vi "Eagle_FPGA Scanner Control.vi"() -> ()   [LabVIEW 2015]
uses:
  <vilib>/Platform/TimedLoop/XDataNode/timing_clust.ctl
  <vilib>/Platform/TimedLoop/XDataNode/nitl_modes.ctl
  <vilib>/Platform/TimedLoop/XDataNode/wakeup.ctl
  <vilib>/rvi/Emulation/niFpgaGetClockAttributes.vi
  <vilib>/rvi/Emulation/niFpgaSctlEmulationGetInTimedLoop.vi
  <vilib>/rvi/Emulation/niFpgaEmulationReportErrorSimple.vi
  <vilib>/rvi/eio/common/nirviEmuTemplateMethod_errors.vi
  <vilib>/rvi/Emulation/niFpgaProcessEmulError.vi
  <vilib>/rvi/Emulation/niFpgaCriticalErrorInLSC.vi
  <vilib>/rvi/FXPMathLib/FxpMul/XNode/nifxpmath_Multiplier.xnode
  <vilib>/eio/EIONode/EIONode.xnode
  <vilib>/rvi/FXPMathLib/FxpAdd/XNode/nifxpmath_Add.xnode
  <vilib>/Platform/TimedLoop/XDataNode/XDataNode.xnode
  <vilib>/rvi/FXPMathLib/sim/FxpSim.dll
  <vilib>/Platform/TimedLoop/XDataNode/XDNodeRunTimeDep.lvlib
  <vilib>/rvi/DataTransferAndStorage/Container/XNode/niFpgaContainer.xnode
  <vilib>/rvi/interface/RandomDataEmulation/nirviRandomDataFpgaMultiElementTemplate.vi
panel:
  in  "One Shot":bool
  in  "Illumination_Ena":bool
  out "Tmp Sens 2":fxp<+,18,3>
  out "Tmp Sens 1":fxp<+,18,3>
  out "X READ 2":fxp<+/-,20,5>
  out "Y READ 2":fxp<+/-,20,5>
  in  "Aim Ctrl":fxp<+,16,3>
  in  "V Range Ctrl":fxp<+,16,3>
  in  "H Range Ctrl":fxp<+,16,3>
  in  "Red Dots Ctrl":fxp<+,16,3>
  in  "LED Ring Ctrl":fxp<+,16,3>
  in  "Y Servo Ena":fxp<+,16,3>
  in  "X Servo Ena":fxp<+,16,3>
  in  "Manual VY":fxp<+/-,20,5>
  in  "Manual VX":fxp<+/-,20,5>
  in  "VX OFFS":fxp<+/-,20,5>
  in  "VY OFFS":fxp<+/-,20,5>
  out "X CMD IND":fxp<+/-,20,5>
  out "Y CMD IND":fxp<+/-,20,5>
  in  "Manual":bool
  in  "NoOfPoints":u16=100
  in  "ScanRate":u32
  in  "Calib Values":T1={"X MULT"=-0.024993896484375, "Y MULT"=-0.033294677734375, "X OFFS"=10.0, "Y OFFS"=10.0}
  in  "NoGO Zone":T2
  in  "Center":cluster{"CX":fxp<+,10,10>, "CY":fxp<+,10,10>}
  in  "NumOfRetries":u16
  out "VX CMD":fxp<+/-,32,17>
  out "VY CMD":fxp<+/-,32,17>
  out "SCAN ENA":bool
  in  "Y Array":fxp<+/-,10,11>[](array[numeric])=[0.0, 0.0, 0.0, 0.0, 0.0, 0.0, 0.0, 0.0, 0.0, 0.0, 0.0, 0.0, 0.0, 0.0, 0.0, 0.0, 0.0, 0.0, 0.0, 0.0, 0.0, 0.0, 0.0, 0.0, 0.0, 0.0, 0.0, 0.0, 0.0, 0.0, 0.0, 0.0, 0.0, 0.0, 0.0, 0.0, 0.0, 0.0, 0.0, 0.0, 0.0, 0.0, 0.0, 0.0, 0.0, 0.0, 0.0, 0.0, 0.0, 0.0, 0.0, 0.0, 0.0, 0.0, 0.0, 0.0, 0.0, 0.0, 0.0, 0.0, 0.0, 0.0, 0.0, 0.0, 0.0, 0.0, 0.0, 0.0, 0.0, 0.0, 0.0, 0.0, 0.0, 0.0, 0.0, 0.0, 0.0, 0.0, 0.0, 0.0, 0.0, 0.0, 0.0, 0.0, 0.0, 0.0, 0.0, 0.0, 0.0, 0.0, 0.0, 0.0, 0.0, 0.0, 0.0, 0.0, 0.0, 0.0, 0.0, 0.0]
  in  "X Array":fxp<+/-,10,11>[](array[numeric])=[0.0, 0.0, 0.0, 0.0, 0.0, 0.0, 0.0, 0.0, 0.0, 0.0, 0.0, 0.0, 0.0, 0.0, 0.0, 0.0, 0.0, 0.0, 0.0, 0.0, 0.0, 0.0, 0.0, 0.0, 0.0, 0.0, 0.0, 0.0, 0.0, 0.0, 0.0, 0.0, 0.0, 0.0, 0.0, 0.0, 0.0, 0.0, 0.0, 0.0, 0.0, 0.0, 0.0, 0.0, 0.0, 0.0, 0.0, 0.0, 0.0, 0.0, 0.0, 0.0, 0.0, 0.0, 0.0, 0.0, 0.0, 0.0, 0.0, 0.0, 0.0, 0.0, 0.0, 0.0, 0.0, 0.0, 0.0, 0.0, 0.0, 0.0, 0.0, 0.0, 0.0, 0.0, 0.0, 0.0, 0.0, 0.0, 0.0, 0.0, 0.0, 0.0, 0.0, 0.0, 0.0, 0.0, 0.0, 0.0, 0.0, 0.0, 0.0, 0.0, 0.0, 0.0, 0.0, 0.0, 0.0, 0.0, 0.0, 0.0]
  in  "Enable":bool
  out "Manual Y IND":fxp<+/-,20,5>
  out "Manual X IND":fxp<+/-,20,5>
  out "Y Servo Rdy":fxp<+,18,3>
  out "X Servo Rdy":fxp<+,18,3>
  out "Y READ":fxp<+/-,20,5>
  out "X READ":fxp<+/-,20,5>
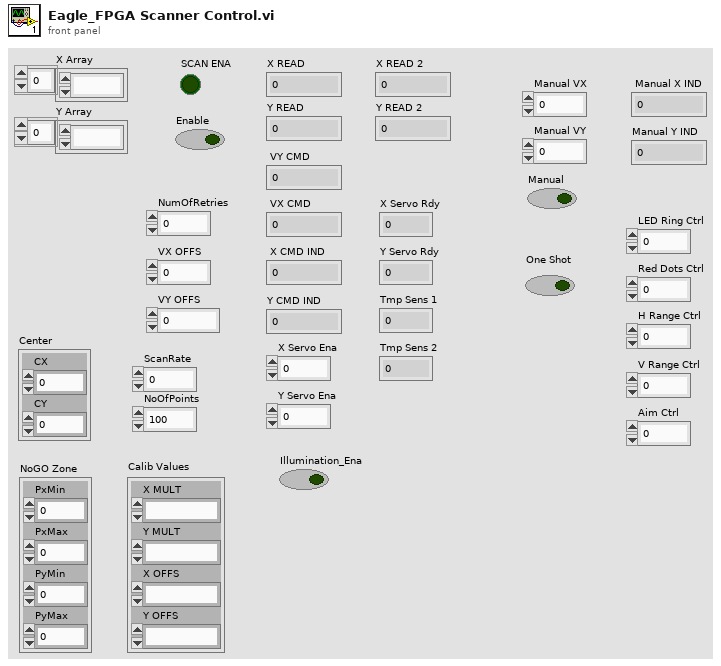
[diagram p1: front panel]
types:
  T1 = cluster{"X MULT":fxp<+/-,20,5>, "Y MULT":fxp<+/-,20,5>, "X OFFS":fxp<+/-,20,5>, "Y OFFS":fxp<+/-,20,5>}
  T2 = cluster{"PxMin":fxp<+,10,10>, "PxMax":fxp<+,10,10>, "PyMin":fxp<+,10,10>, "PyMax":fxp<+,10,10>}
  T3 = typedef "XDNodeRunTimeDep.lvlib/timing_clust.ctl" = cluster{"Expected End [f-1]":u64, "Actual End [f-1]":u64, "Finished Late? [f-1]":bool, "Expected End [i-1]":u64, "Actual End [i-1]":u64, "Finished Late? [i-1]":bool, "Expected Start [i]":u64, "Actual Start [i]":u64, "Expected Start [f]":u64, "Actual Start [f]":u64, "Source Name":string, "Structure Name":string, "Period":i64, "Deadline":i64, "Offset":i64, "Start":i64, "Priority":i32, "Timeout":i32, "Mode":T4, "Wakeup Reason":T5, "Error":errorcluster, "Source Type":string, "Secondary Source Type":string, "Global End Time":u64, "Global Start Time":u64, "Frame Duration":u64, "Iteration Duration":u64, "Assigned CPU":i32, "I/O Scan Engine Mode":u32}
  T4 = typedef "XDNodeRunTimeDep.lvlib/nitl_modes.ctl" = enum32{"No Change", "Process missed periods, maintain original phase", "Discard missed periods, maintain original phase", "Process missed periods, ignore original phase", "Discard missed periods, ignore original phase"}
  T5 = typedef "XDNodeRunTimeDep.lvlib/wakeup.ctl" = enum32{"Normal", "Aborted", "Asynchronous wakeup", "Timing source error", "Timed loop error", "Timeout"}
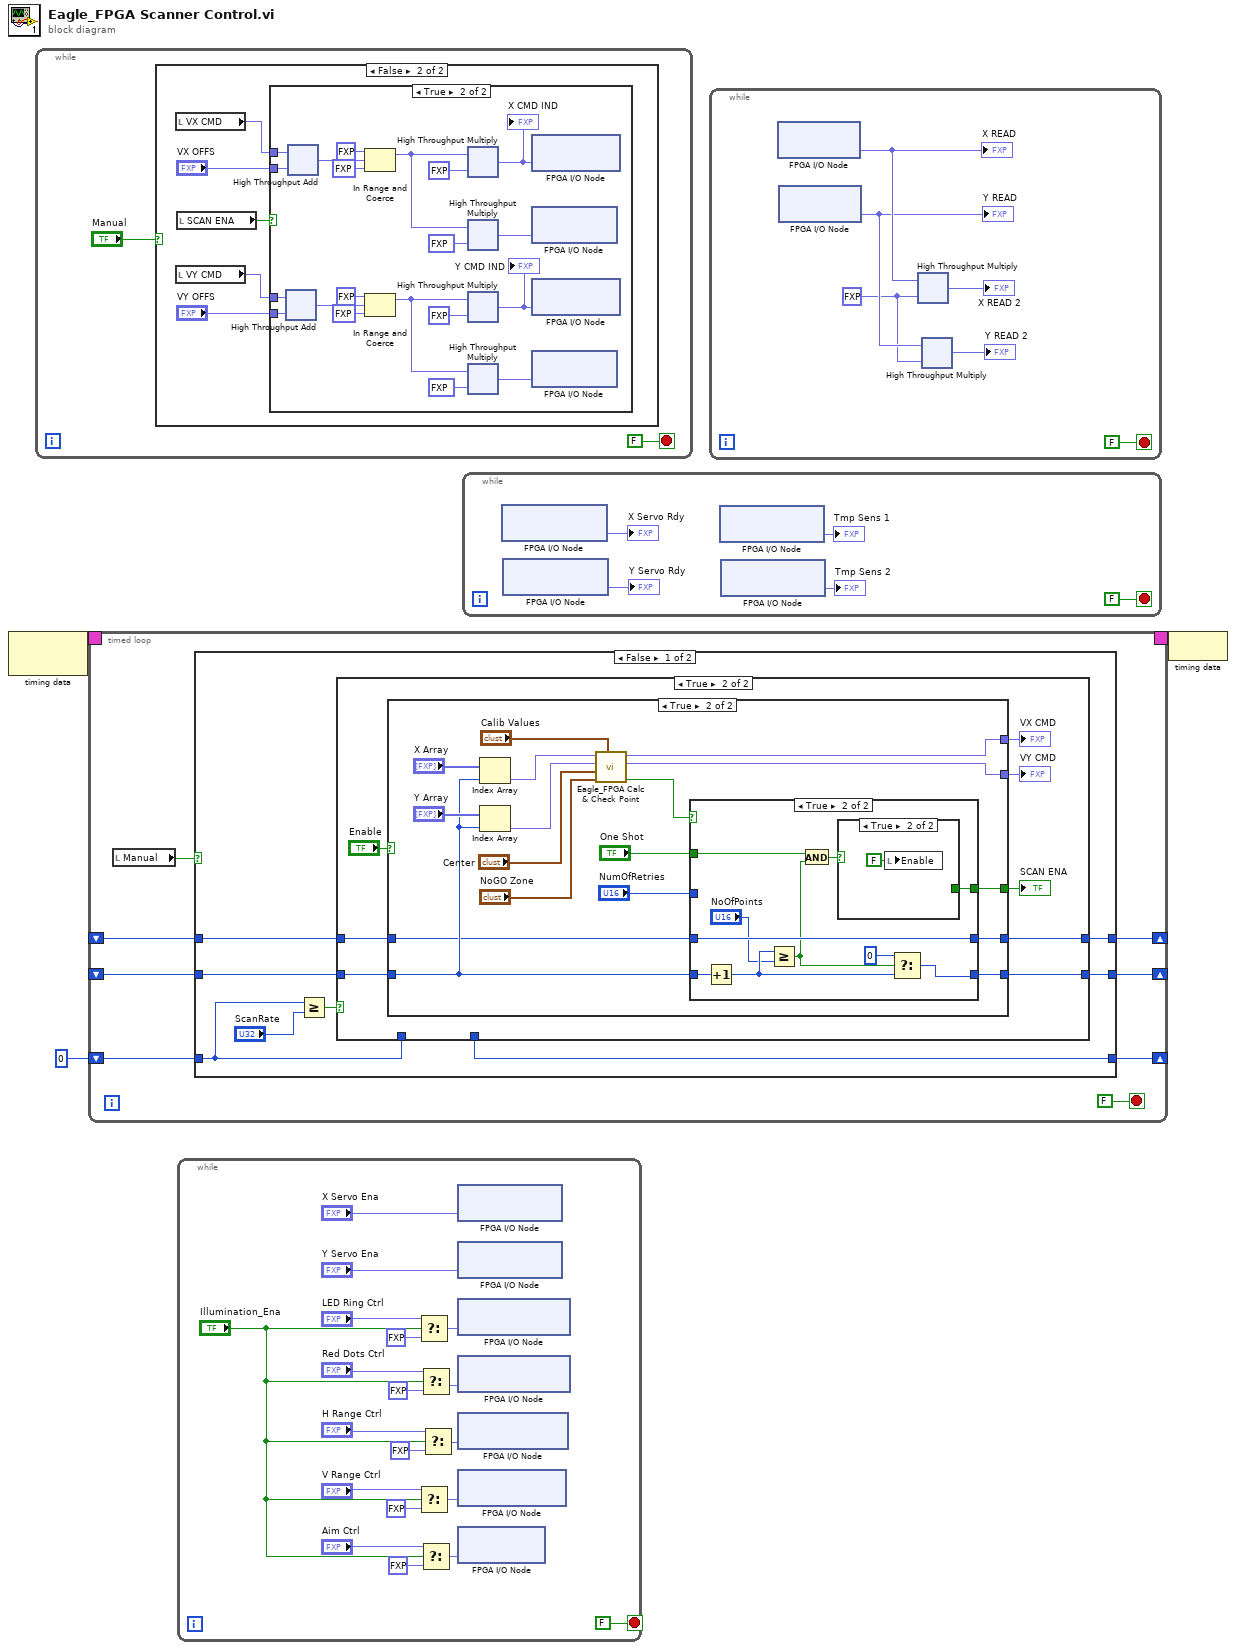
[diagram p0: block diagram]
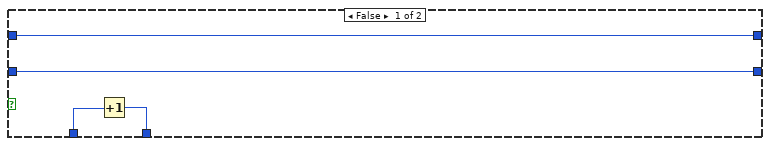
[diagram p2: hidden frame]
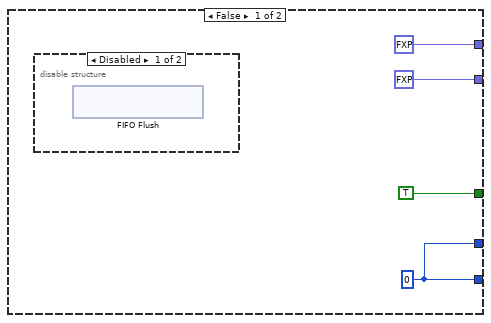
[diagram p3: hidden frame]
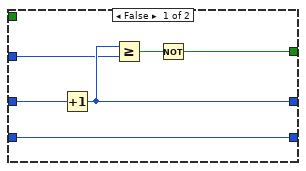
[diagram p5: hidden frame]
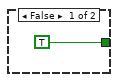
[diagram p6: hidden frame]
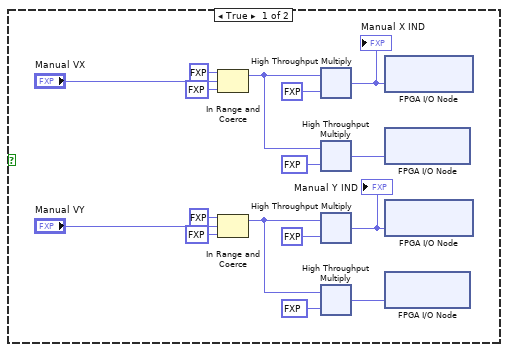
[diagram p8: hidden frame]
diagram:
  n1 = node-c288() -> (w3:T3)  [unwired: 1 in]
  n2 = while {
    stop <- FALSE stop-if-true
    n3 = case shown="False" "Manual" {
      frame True {
        n4 = In Range and Coerce(upper limit=fxp<+/-,20,5> 10.0, x="Manual VX", lower limit=fxp<+/-,20,5> -10.0 ("upper limit")) -> (coerced(x)=w13:fxp<+/-,20,5>)  [unwired: 1 out]
        n5 = In Range and Coerce(upper limit=fxp<+/-,20,5> 10.0, x="Manual VY", lower limit=fxp<+/-,20,5> -10.0 ("upper limit")) -> (coerced(x)=w8:fxp<+/-,20,5>)  [unwired: 1 out]
        n6 = xnode ("High Throughput Multiply")("x"=w13, "y"=fxp<+/-,20,5> 0.5) -> ("x*y"=w19:fxp<+/-,20,5>)
        "Manual X IND" <- w19
        n7 = xnode ("High Throughput Multiply")("x"=w13, "y"=fxp<+/-,20,5> -0.5) -> ("x*y"=w17:fxp<+/-,20,5>)
        n8 = xnode ("High Throughput Multiply")("x"=w8, "y"=fxp<+/-,20,5> 0.5) -> ("x*y"=w15:fxp<+/-,20,5>)
        "Manual Y IND" <- w15
        n9 = xnode ("High Throughput Multiply")("x"=w8, "y"=fxp<+/-,20,5> -0.5) -> ("x*y"=w14:fxp<+/-,20,5>)
        n10 = xnode "FPGA I/O Node"("X CMD+"=w19) -> ()  [unwired: 1 in, 1 out]
        n11 = xnode "FPGA I/O Node"("X CMD-"=w17) -> ()  [unwired: 1 in, 1 out]
        n12 = xnode "FPGA I/O Node"("Y CMD+"=w15) -> ()  [unwired: 1 in, 1 out]
        n13 = xnode "FPGA I/O Node"("Y CMD-"=w14) -> ()  [unwired: 1 in, 1 out]
      }
      frame False {
        n14 = local read "VX CMD"() -> (w23:fxp<+/-,32,17>)
        n15 = local read "VY CMD"() -> (w22:fxp<+/-,32,17>)
        n16 = local read "SCAN ENA"() -> (w24:bool)
        n17 = case shown="True" w24 {
          tunnel: "VX OFFS" -> [_ w38]
          tunnel: "VY OFFS" -> [_ w37]
          tunnel: w23 -> [_ w28]
          tunnel: w22 -> [_ w27]
          frame False {
          }
          frame True {
            n18 = xnode ("High Throughput Add")("x"=w27, "y"=w37) -> ("x+y"=w30:fxp<+/-,33,18>)
            n19 = xnode ("High Throughput Add")("x"=w28, "y"=w38) -> ("x+y"=w36:fxp<+/-,33,18>)
            n20 = In Range and Coerce(upper limit=fxp<+/-,20,5> 10.0, x=w36, lower limit=fxp<+/-,20,5> -10.0 ("upper limit")) -> (coerced(x)=w35:fxp<+/-,33,18>)  [unwired: 1 out]
            n21 = In Range and Coerce(upper limit=fxp<+/-,20,5> 10.0, x=w30, lower limit=fxp<+/-,20,5> -10.0 ("upper limit")) -> (coerced(x)=w29:fxp<+/-,33,18>)  [unwired: 1 out]
            n22 = xnode ("High Throughput Multiply")("x"=w35, "y"=fxp<+/-,20,5> 0.5) -> ("x*y"=w44:fxp<+/-,20,5>)
            "X CMD IND" <- w44
            n23 = xnode ("High Throughput Multiply")("x"=w35, "y"=fxp<+/-,20,5> -0.5) -> ("x*y"=w42:fxp<+/-,20,5>)
            n24 = xnode ("High Throughput Multiply")("x"=w29, "y"=fxp<+/-,20,5> 0.5) -> ("x*y"=w40:fxp<+/-,20,5>)
            "Y CMD IND" <- w40
            n25 = xnode ("High Throughput Multiply")("x"=w29, "y"=fxp<+/-,20,5> -0.5) -> ("x*y"=w39:fxp<+/-,20,5>)
            n26 = xnode "FPGA I/O Node"("X CMD+"=w44) -> ()  [unwired: 1 in, 1 out]
            n27 = xnode "FPGA I/O Node"("X CMD-"=w42) -> ()  [unwired: 1 in, 1 out]
            n28 = xnode "FPGA I/O Node"("Y CMD+"=w40) -> ()  [unwired: 1 in, 1 out]
            n29 = xnode "FPGA I/O Node"("Y CMD-"=w39) -> ()  [unwired: 1 in, 1 out]
          }
        }
      }
    }
  }
  n30 = timed-loop {
    timing: w3 -> [_]
    timing-out: [_] -> w2
    shift-right: [w50] -> _
    shift-left: _ -> [w53]
    shift-right: [w52] -> _
    shift-left: _ -> [w51]
    shift-right: [w49] -> _
    shift-left: u32 0 -> [w48]
    stop <- FALSE stop-if-true
    n31 = local read "Manual"() -> (w47:bool)
    n32 = case shown="False" w47 {
      tunnel: w53 -> [w62 w115]
      tunnel: [w61 w116] -> w52
      tunnel: w51 -> [w60 w116]
      tunnel: [w59 w115] -> w50
      tunnel: [w57 w114] -> w49
      tunnel: w48 -> [w56 w114]
      frame False {
        n33 = Greater Or Equal?(x=w56, y="ScanRate") -> (x >= y?=w58:bool)
        n34 = case shown="True" w58 {
          tunnel: w62 -> [w65 w73]
          tunnel: [w66 w69] -> w61
          tunnel: w60 -> [w66 w68]
          tunnel: [w65 w67] -> w59
          tunnel: w56 -> [w64 _]
          tunnel: [w63 _] -> w57
          frame False {
            n35 = Increment(x=w64) -> (x+1=w63:u32)
          }
          frame True {
            n36 = case shown="True" "Enable" {
              tunnel: w73 -> [_ w89]
              tunnel: [fxp<+/-,20,5> 10.0 ("VX CMD") w91] -> w72
              tunnel: [fxp<+/-,20,5> 10.0 ("VY CMD") w90] -> w71
              tunnel: [TRUE ("SCAN ENA") w84] -> w70
              tunnel: [w75 w86] -> w69
              tunnel: w68 -> [_ w87]
              tunnel: [w75 w88] -> w67
              frame False {
                w75 = u16 0
                n37 = disable-structure shown="Disabled" {
                  frame Disabled {
                    n38 = xnode ("FIFO Flush")() -> ()  [unwired: 1 in, 1 out]
                  }
                  frame Enabled {
                  }
                }
              }
              frame True {
                n39 = Index Array(array="X Array", index=w89) -> (element=w93:fxp<+/-,10,11>)
                n40 = Index Array(array="Y Array", index=w89) -> (element=w92:fxp<+/-,10,11>)
                n41 = call "Eagle_FPGA Calc & Check Point.vi"("Calib Values"="Calib Values", "NoGO Zone"="NoGO Zone", "Center"="Center", "PX"=w92, "PY"=w93) -> ("SCAN ENA"=w79:bool, "VY CMD"=w90:fxp<+/-,32,17>, "VX CMD"=w91:fxp<+/-,32,17>)  [unwired: 4 in]
                n42 = case shown="True" w79 {
                  tunnel: w89 -> [w101 w111]
                  tunnel: [w101 w109] -> w88
                  tunnel: w87 -> [w100 w110]
                  tunnel: [w99 w110] -> w86
                  tunnel: "NumOfRetries" -> [w98 _]
                  tunnel: [w96 w105] -> w84
                  tunnel: "One Shot" -> [_ w104]
                  frame False {
                    n43 = Increment(x=w100) -> (x+1=w99:u16)
                    n44 = Greater Or Equal?(x=w99, y=w98) -> (x >= y?=w97:bool)
                    n45 = Not(x=w97) -> (.not. x?=w96:bool)
                  }
                  frame True {
                    n46 = Increment(x=w111) -> (x+1=w107:u16)
                    n47 = Greater Or Equal?(x=w107, y="NoOfPoints") -> (x >= y?=w103:bool)
                    n48 = And(x=w104, y=w103) -> (x .and. y?=w102:bool)
                    n49 = case shown="True" w102 {
                      tunnel: [TRUE _] -> w105
                      frame False {
                      }
                      frame True {
                        n50 = local write "Enable"(FALSE ("Reset")) -> ()
                      }
                    }
                    n51 = Select(t=u16 0, s=w103, f=w107) -> (s? t:f=w109:u16)
                  }
                }
              }
            }
            "SCAN ENA" <- w70
            "VY CMD" <- w71
            "VX CMD" <- w72
          }
        }
      }
      frame True {
      }
    }
  }
  n52 = while {
    stop <- FALSE stop-if-true
    n53 = Select(t="LED Ring Ctrl", s="Illumination_Ena", f=fxp<+,16,3> 0.0) -> (s? t:f=w124:fxp<+,16,3>)
    n54 = Select(t="V Range Ctrl", s="Illumination_Ena", f=fxp<+,16,3> 5.0) -> (s? t:f=w130:fxp<+,16,3>)
    n55 = Select(t="Red Dots Ctrl", s="Illumination_Ena", f=fxp<+,16,3> 0.0) -> (s? t:f=w126:fxp<+,16,3>)
    n56 = Select(t="Aim Ctrl", s="Illumination_Ena", f=fxp<+,16,3> 5.0) -> (s? t:f=w134:fxp<+,16,3>)
    n57 = Select(t="H Range Ctrl", s="Illumination_Ena", f=fxp<+,16,3> 5.0) -> (s? t:f=w128:fxp<+,16,3>)
    n58 = xnode "FPGA I/O Node"("X Servo Ena"="X Servo Ena") -> ()  [unwired: 1 in, 1 out]
    n59 = xnode "FPGA I/O Node"("Y Servo Ena"="Y Servo Ena") -> ()  [unwired: 1 in, 1 out]
    n60 = xnode "FPGA I/O Node"("LED Ring Ctrl"=w124) -> ()  [unwired: 1 in, 1 out]
    n61 = xnode "FPGA I/O Node"("Red Dots Ctrl"=w126) -> ()  [unwired: 1 in, 1 out]
    n62 = xnode "FPGA I/O Node"("H Range Ctrl"=w128) -> ()  [unwired: 1 in, 1 out]
    n63 = xnode "FPGA I/O Node"("V Range Ctrl"=w130) -> ()  [unwired: 1 in, 1 out]
    n64 = xnode "FPGA I/O Node"("Aim Ctrl"=w134) -> ()  [unwired: 1 in, 1 out]
  }
  n65 = while {
    stop <- FALSE stop-if-true
    n66 = xnode "FPGA I/O Node"() -> ("X Servo Rdy"=→"X Servo Rdy":fxp<+,18,3>)  [unwired: 1 in, 1 out]
    n67 = xnode "FPGA I/O Node"() -> ("Y Servo Rdy"=→"Y Servo Rdy":fxp<+,18,3>)  [unwired: 1 in, 1 out]
    n68 = xnode "FPGA I/O Node"() -> ("Tmp Sens 1"=→"Tmp Sens 1":fxp<+,18,3>)  [unwired: 1 in, 1 out]
    n69 = xnode "FPGA I/O Node"() -> ("Tmp Sens 2"=→"Tmp Sens 2":fxp<+,18,3>)  [unwired: 1 in, 1 out]
  }
  n70 = while {
    stop <- FALSE stop-if-true
    w143 = fxp<+/-,20,5> 2.0 ("Y READ")
    n71 = xnode "FPGA I/O Node"() -> ("X READ"=w145:fxp<+/-,20,5>)  [unwired: 1 in, 1 out]
    "X READ" <- w145
    n72 = xnode "FPGA I/O Node"() -> ("Y READ"=w144:fxp<+/-,20,5>)  [unwired: 1 in, 1 out]
    "Y READ" <- w144
    n73 = xnode ("High Throughput Multiply")("x"=w145, "y"=w143) -> ("x*y"=→"X READ 2":fxp<+/-,20,5>)
    n74 = xnode ("High Throughput Multiply")("x"=w144, "y"=w143) -> ("x*y"=→"Y READ 2":fxp<+/-,20,5>)
  }
  n75 = node-c288(w2) -> ()
